vi "Get Additional data.vi"(11 "Additional Data":variant) -> (3 "Formated Additional data":string)   [LabVIEW 2025]
doc: "Converting data from Variant to defined data types and converting them to Formated string.\nPossible formats CAN message, Number, Array of numbers, String"
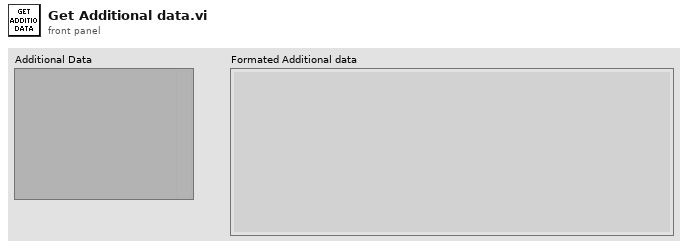
[diagram p1: front panel]
types:
  T1 = cluster{"ID":u32, "MSGTYPE":u8, "LEN":u8, "DATA[0]":u8, "DATA[1]":u8, "DATA[2]":u8, "DATA[3]":u8, "DATA[4]":u8, "DATA[5]":u8, "DATA[6]":u8, "DATA[7]":u8}[]
  T2 = cluster{"ID":u32, "MSGTYPE":u8, "LEN":u8, "DATA[0]":u8, "DATA[1]":u8, "DATA[2]":u8, "DATA[3]":u8, "DATA[4]":u8, "DATA[5]":u8, "DATA[6]":u8, "DATA[7]":u8}
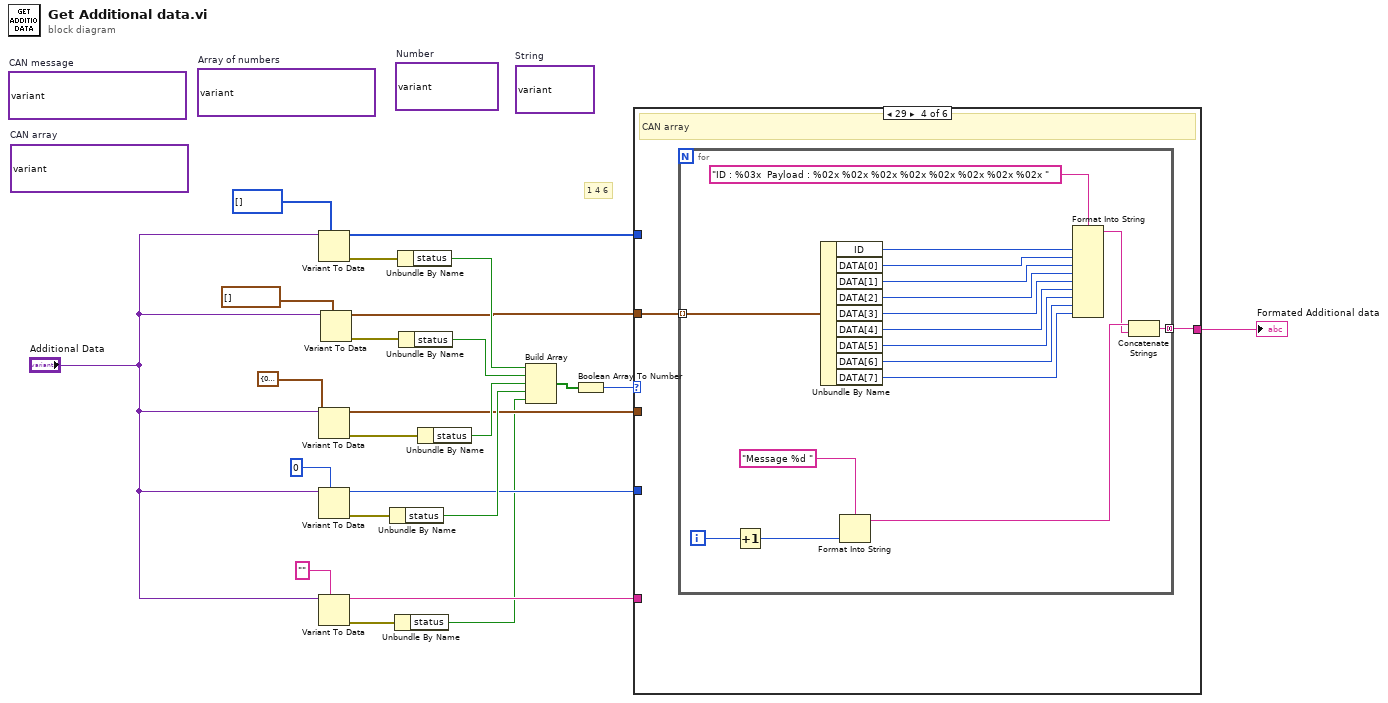
[diagram p0: block diagram]
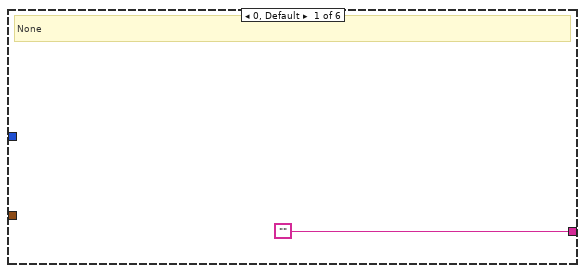
[diagram p2: hidden frame]
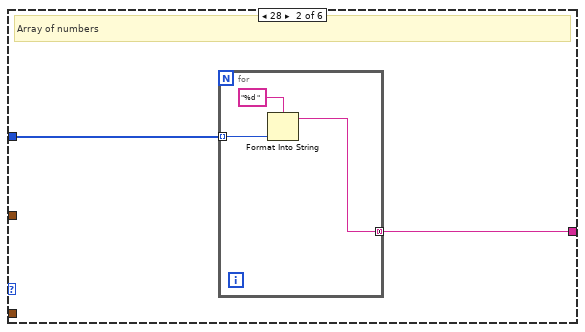
[diagram p3: hidden frame]
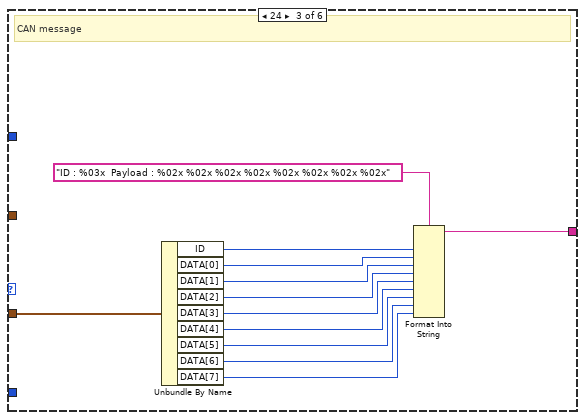
[diagram p4: hidden frame]
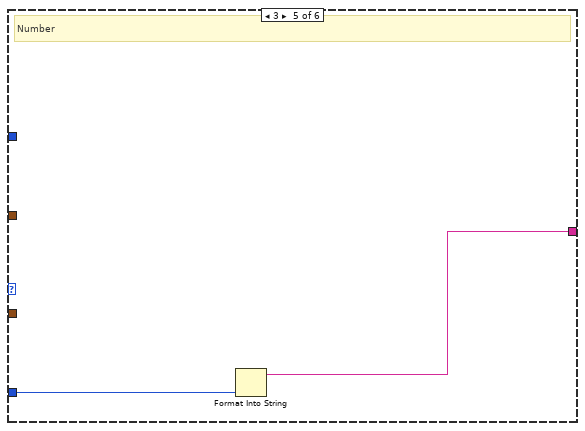
[diagram p5: hidden frame]
diagram:
  (unwired) variant  # CAN array
  (unwired) variant  # String
  (unwired) variant  # Number
  (unwired) variant  # Array of numbers
  (unwired) variant  # CAN message
  # "1 4 6"
  n1 = Variant To Data(type=i32[] [], Variant="Additional Data") -> (data=w12:i32[], error out=w21:errorcluster)  [unwired: 1 in]
  n2 = Variant To Data(type=T2 {"ID"=0, "MSGTYPE"=0, "LEN"=0, "DATA[0]"=0, "DATA[1]"=0, "DATA[2]"=0, "DATA[3]"=0, "DATA[4]"=0, "DATA[5]"=0, "DATA[6]"=0, "DATA[7]"=0} ("MessageBuffer out"), Variant="Additional Data") -> (data=w13:T2, error out=w20:errorcluster)  [unwired: 1 in]
  n3 = Variant To Data(type=0, Variant="Additional Data") -> (data=w14:i32, error out=w19:errorcluster)  [unwired: 1 in]
  n4 = Variant To Data(type="", Variant="Additional Data") -> (data=w8:string, error out=w10:errorcluster)  [unwired: 1 in]
  n5 = Variant To Data(type=T1 [] ("MessageBuffer out"), Variant="Additional Data") -> (data=w2:T1, error out=w5:errorcluster)  [unwired: 1 in]
  n6 = Unbundle By Name(w19) -> ("status"=w17:bool)
  n7 = Unbundle By Name(w10) -> ("status"=w7:bool)
  n8 = Unbundle By Name(w21) -> ("status"=w4:bool)
  n9 = Unbundle By Name(w5) -> ("status"=w3:bool)
  n10 = Unbundle By Name(w20) -> ("status"=w18:bool)
  n11 = Build Array(w4, w3, w18, w17, w7) -> (w16:bool[])
  n12 = Boolean Array To Number(Boolean array=w16) -> (number=w15:u32)
  n13 = case shown="29" w15 {
    tunnel: w14 -> [_ _ _ _ w63 _]
    tunnel: w13 -> [_ _ w31 _ _ _]
    tunnel: w12 -> [_ w27 _ _ _ _]
    tunnel: ["" w26 w32 w44 w62 w64] -> w11
    tunnel: w8 -> [_ _ _ _ _ w64]
    tunnel: w2 -> [_ _ _ w43 _ _]
    frame 0, Default {
      # "None"
    }
    frame 28 {
      # "Array of numbers"
      n14 = for {
        tunnel: w27 -> [w30] mode=indexing
        tunnel: [w28] -> w26 mode=concatenating
        n15 = Format Into String(format string="%d ", w30) -> (resulting string=w28:string)  [unwired: 2 in, 1 out]
      }
    }
    frame 24 {
      # "CAN message"
      n16 = Unbundle By Name(w31) -> ("ID"=w41:u32, "DATA[0]"=w40:u8, "DATA[1]"=w39:u8, "DATA[2]"=w38:u8, "DATA[3]"=w37:u8, "DATA[4]"=w36:u8, "DATA[5]"=w35:u8, "DATA[6]"=w34:u8, "DATA[7]"=w33:u8)
      n17 = Format Into String(format string="ID : %03x  Payload : %02x %02x %02x %02x %02x %02x %02x %02x", w41, w40, w39, w38, w37, w36, w35, w34, w33) -> (resulting string=w32:string)  [unwired: 2 in, 1 out]
    }
    frame 29 {
      # "CAN array"
      n18 = for {
        tunnel: [w46] -> w44 mode=concatenating
        tunnel: w43 -> [w45] mode=indexing
        i -> [w51]
        n19 = Increment(x=w51) -> (x+1=w49:i32)
        n20 = Unbundle By Name(w45) -> ("ID"=w60:u32, "DATA[0]"=w59:u8, "DATA[1]"=w58:u8, "DATA[2]"=w57:u8, "DATA[3]"=w56:u8, "DATA[4]"=w55:u8, "DATA[5]"=w54:u8, "DATA[6]"=w53:u8, "DATA[7]"=w52:u8)
        n21 = Format Into String(format string="Message %d ", w49) -> (resulting string=w48:string)  [unwired: 2 in, 1 out]
        n22 = Format Into String(format string="ID : %03x  Payload : %02x %02x %02x %02x %02x %02x %02x %02x ", w60, w59, w58, w57, w56, w55, w54, w53, w52) -> (resulting string=w47:string)  [unwired: 2 in, 1 out]
        n23 = Concatenate Strings(w48, w47) -> (w46:string)
      }
    }
    frame 3 {
      # "Number"
      n24 = Format Into String(w63) -> (resulting string=w62:string)  [unwired: 3 in, 1 out]
    }
    frame 11 {
      # "String data"
    }
  }
  "Formated Additional data" <- w11
